vi "Tree.vi"   [LabVIEW 2011, in "Tinkerforge.lvlib"]
doc: "This VI shows all Top-Level VIs."
uses:
  Tinkerforge.lvlib
  Classes/IP Connection/IP Connection.lvclass
  Classes/Ambient Light Bricklet/Ambient Light Bricklet.lvclass
  Classes/Humidity Bricklet/Humidity Bricklet.lvclass
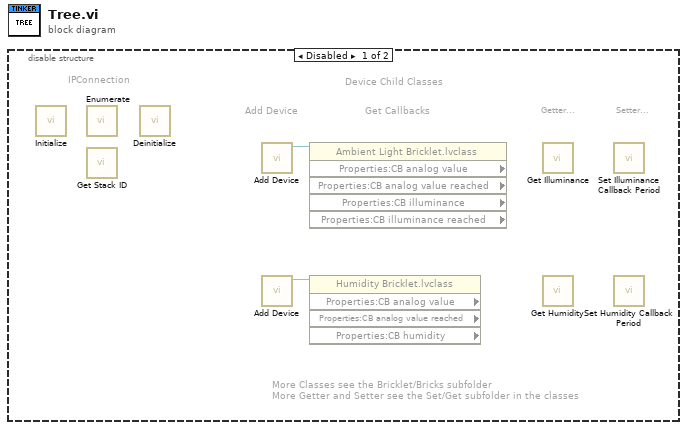
[diagram p0: block diagram]
diagram:
  n1 = disable-structure shown="Disabled" {
    frame Disabled {
      # "More Classes see the Bricklet/Bricks subfolder\nMore Getter and Setter see the Set/Get subfolder in the classes"
      # "Setter..."
      # "Getter..."
      # "Get Callbacks"
      # "Add Device"
      # "Device Child Classes"
      # "IPConnection"
      n2 = call "Initialize.vi"() -> ()  [unwired: 10 in, 2 out]
      n3 = call "Enumerate.vi"() -> ()  [unwired: 10 in, 2 out]
      n4 = call "Get Stack ID.vi"() -> ()  [unwired: 7 in, 5 out]
      n5 = call "Deinitialize.vi"() -> ()  [unwired: 11 in, 1 out]
      n6 = call "Add Device.vi"() -> ("Ambient Light Bricklet"=w2:refnum<class "Ambient Light Bricklet.lvclass">)  [unwired: 10 in, 1 out]
      n7 = call "Add Device.vi"() -> ("Humidity Bricklet"=w1:refnum<class "Humidity Bricklet.lvclass">)  [unwired: 10 in, 1 out]
      n8 = property class="Ambient Light Bricklet.lvclass" props=["Properties:CB analog value", "Properties:CB analog value reached", "Properties:CB illuminance", "Properties:CB illuminance reached"](reference=w2) -> ()  [unwired: 1 in, 6 out]
      n9 = property class="Humidity Bricklet.lvclass" props=["Properties:CB analog value", "Properties:CB analog value reached", "Properties:CB humidity"](reference=w1) -> ()  [unwired: 1 in, 5 out]
      n10 = call "Get Illuminance.vi"() -> ()  [unwired: 9 in, 3 out]
      n11 = call "Get Humidity.vi"() -> ()  [unwired: 9 in, 3 out]
      n12 = call "Set Illuminance Callback Period.vi"() -> ()  [unwired: 10 in, 2 out]
      n13 = call "Set Humidity Callback Period.vi"() -> ()  [unwired: 10 in, 2 out]
    }
    frame Enabled {
    }
  }
